vi "Set Request Tick.vi"(8 "error in":errorcluster, 10 "Request Tick":u32, 11 "Check if Confirmed Msg in":refnum<class "Check if Confirmed Msg.lvclass">) -> (0 "error out":errorcluster, 3 "Check if Confirmed Msg out":refnum<class "Check if Confirmed Msg.lvclass">)   [LabVIEW 2020, in "CANopen.lvlib" / "Network Management.lvlib" / "Node Guard.lvlib" / "Check if Confirmed Msg.lvclass"]
uses:
  Check if Confirmed Msg.lvclass
  Check if Confirmed Msg.lvclass/Check if Confirmed Msg.ctl
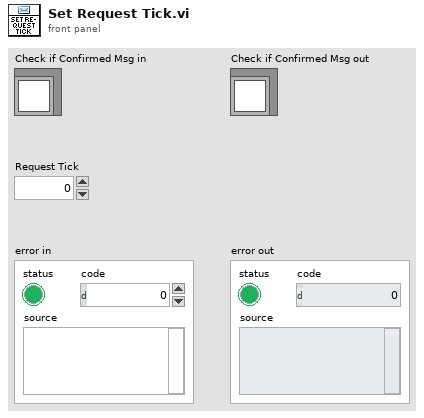
[diagram p1: front panel]
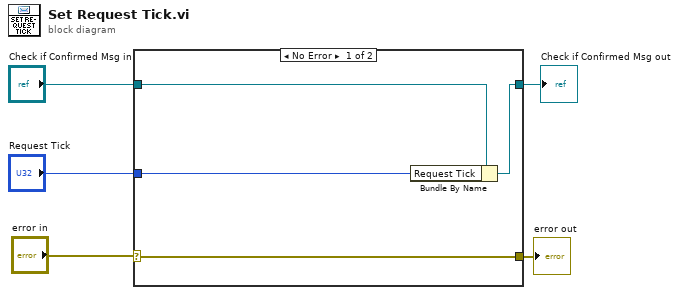
[diagram p0: block diagram]
diagram:
  n1 = case shown="No Error" "error in" {
    selector: "error in" -> [w9 w10]
    tunnel: [w9 w10] -> w2
    tunnel: [w7 w11] -> w4
    tunnel: "Check if Confirmed Msg in" -> [w8 w11]
    tunnel: "Request Tick" -> [w6 _]
    frame No Error {
      n2 = Bundle By Name(cluster=w8, "Request Tick"=w6) -> (w7:refnum<class "Check if Confirmed Msg.lvclass">)
    }
    frame Error {
    }
  }
  "error out" <- w2
  "Check if Confirmed Msg out" <- w4
